vi "Compare Optimiser Cells.vi"(1 "Optimieser Cell B":refnum<class "Optimiser Cell.lvclass">, 2 "Optimieser Cell A":refnum<class "Optimiser Cell.lvclass">) -> (0 "Equal":bool)   [LabVIEW 2020, in "TALOS.lvlib" / "Run Utilities.lvlib" / "Optimiser Cell.lvclass"]
doc: "Compare if the two optimisation cells refer to the same optimisation process"
uses:
  Optimiser Cell.lvclass
  Optimiser Cell.lvclass/Optimiser Cell.ctl
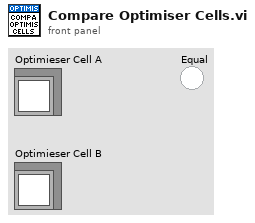
[diagram p1: front panel]
types:
  T1 = typedef "TALOS.lvlib/Run Utilities.lvlib/Optimiser Cell.lvclass/Optimisation observable.ctl" = cluster{"Name":string, "Weight":dbl}
  T2 = typedef "TALOS.lvlib/Run Utilities.lvlib/Optimiser Cell.lvclass/Optimisation Strategy.ctl" = enum16{"Maximize", "Minimize", "Value"}
  T3 = cluster{"Kasli Name":string, "Script Path":path, "Script Parameters":string[], "Observables":T1[], "Optimisation Strategy":T2, "Optimisation Strategy Value":dbl, "Paramters - Numeric":cluster{"Name":string, "From":dbl, "To":dbl, "dtype":enum16{"INT", "DBL"}}[], "Parameters - string":cluster{"Name":string, "sorted array":string[]}[]}
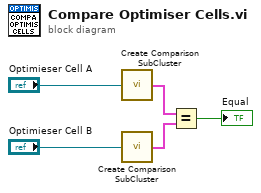
[diagram p0: block diagram]
diagram:
  n1 = call "Create Comparison SubCluster.vi"("Optimiser Cell in"="Optimieser Cell A") -> ("Cluster"=w4:T3)
  n2 = call "Create Comparison SubCluster.vi"("Optimiser Cell in"="Optimieser Cell B") -> ("Cluster"=w1:T3)
  n3 = Equal?(x=w4, y=w1) -> (x = y?=→"Equal":bool)
